vi "IMAQ Mask.vi"() -> ()   [LabVIEW 2012, in "LightPipes.lvlib"]
uses:
  LightPipes.lvlib
  <vilib>/vision/NI_Vision_Development_Module.lvlib
panel:
  in  "Image Type":u32(ring)=1 items=["8 bits", "16 bits", "Float", "Complex", "RGB", "HSL"]
  in  "Noise Value":i32
  in  "Noise Remove":bool
  in  "Save":bool
  in  "Input Image Path":path
  out "Image":T1(plugin-control)
  in  "Stop":bool
  in  "Mask":bool
  out "Mask":T1(plugin-control)
  # "1. Select the Image File\n2. Select the Region of Interest (ROI)\n3. Press Mask\n4. Press Save to save the masked picture\n5. Press Return to exit"
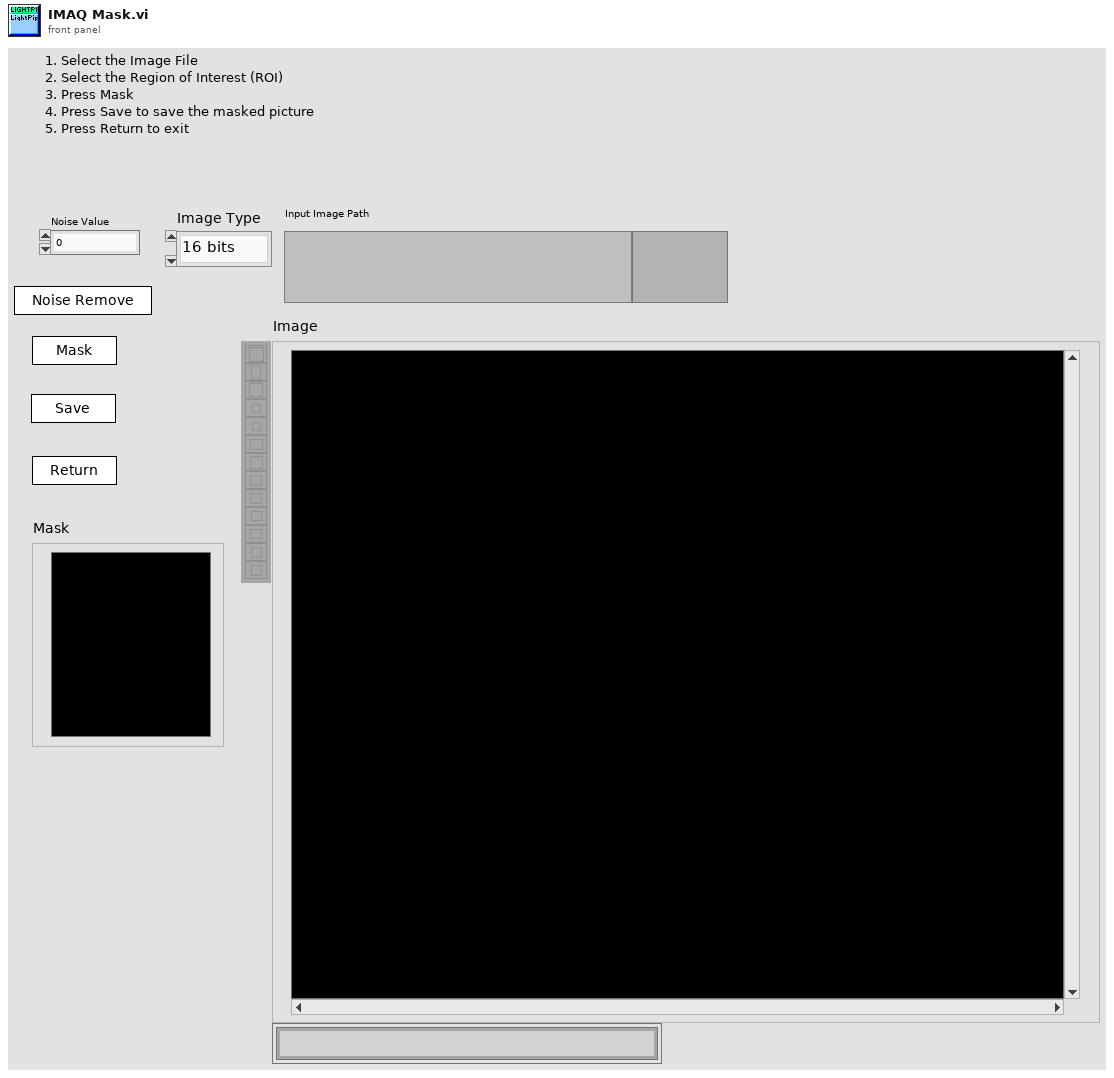
[diagram p1: front panel]
types:
  T1 = typedef "IMAQ Image.ctl" = refnum<image>
  T2 = cluster{"Global Rectangle":i32[], "Contours":cluster{"Contour Type":u32, "ROI Type":u32, "Points":i32[]}[]}
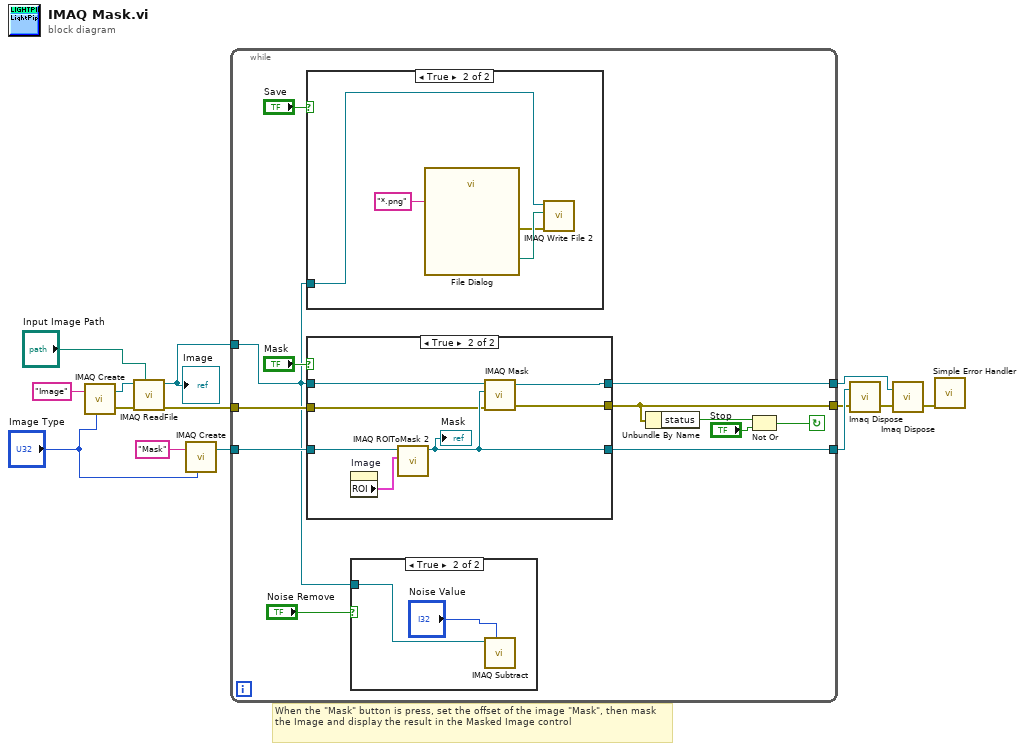
[diagram p0: block diagram]
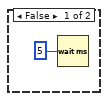
[diagram p3: hidden frame]
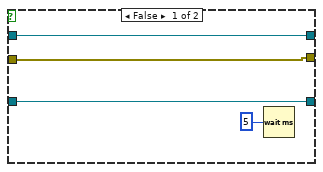
[diagram p4: hidden frame]
diagram:
  # "When the \"Mask\" button is press, set the offset of the image \"Mask\", then mask the Image and display the result in the Masked Image control"
  n1 = call "IMAQ Create"("Image Name"="Image", "Image Type"="Image Type") -> ("New Image"=w8:T1, "error out"=w13:errorcluster)  [unwired: 2 in, 1 out]
  n2 = call "IMAQ ReadFile"("File Path"="Input Image Path", "error in (no error)"=w13, "Image"=w8) -> ("error out"=w12:errorcluster, "Image Out"=w2:T1)  [unwired: 2 in, 5 out]
  "Image" <- w2
  n3 = call "IMAQ Create"("Image Name"="Mask", "Image Type"="Image Type") -> ("New Image"=w9:T1)  [unwired: 2 in, 2 out]
  n4 = while {
    tunnel: w2 -> [w15]
    tunnel: w12 -> [w25]
    tunnel: [w24] -> w3
    tunnel: [w18] -> w7
    tunnel: [w20] -> w5
    tunnel: w9 -> [w16]
    stop <- w21 continue-if-true
    n5 = case shown="True" "Save" {
      tunnel: w15 -> [_ w31]
      frame False {
        n6 = Wait (ms)(milliseconds to wait=u32 5) -> ()  [unwired: 1 out]
      }
      frame True {
        n7 = call "File Dialog"("pattern (all files)"="*.png") -> ("selected path"=w33:path, "error out"=w30:errorcluster)  [unwired: 11 in, 2 out]
        n8 = call-poly "IMAQ Write File 2"("error in (no error)"=w30, "File Path"=w33, "Image"=w31) -> ()  [unwired: 7 in, 2 out]
      }
    }
    n9 = case shown="True" "Mask" {
      tunnel: w15 -> [w37 w44]
      tunnel: w25 -> [w36 w40]
      tunnel: [w37 w38] -> w18
      tunnel: [w36 w43] -> w24
      tunnel: [w34 w41] -> w20
      tunnel: w16 -> [w34 w39]
      frame False {
        n10 = Wait (ms)(milliseconds to wait=u32 5) -> ()  [unwired: 1 out]
      }
      frame True {
        n11 = property on="Image" class="ImageControl"() -> ("ROI"=w42:T2)  [unwired: 2 in, 2 out]
        n12 = call "IMAQ ROIToMask 2"("ROI Descriptor"=w42, "Image"=w39) -> ("Image Out"=w41:T1)  [unwired: 7 in, 2 out]
        "Mask" <- w41
        n13 = call "IMAQ Mask"("error in (no error)"=w40, "Image Mask"=w41, "Image Src"=w44) -> ("error out"=w43:errorcluster, "Image Dst Out"=w38:T1)  [unwired: 1 in, 1 out]
      }
    }
    n14 = case shown="True" "Noise Remove" {
      tunnel: w15 -> [_ w28]
      frame False {
      }
      frame True {
        n15 = call "IMAQ Subtract"("Image Src A"=w28, "Constant"="Noise Value") -> ()  [unwired: 5 in, 2 out]
      }
    }
    n16 = Unbundle By Name(w24) -> ("status"=w23:bool)
    n17 = Not Or(1:"Stop", 2:w23) -> (0:w21:bool)
  }
  n18 = call "Imaq Dispose"("Image"=w5, "error in (no error)"=w3) -> ("error out"=w4:errorcluster)  [unwired: 1 in, 3 out]
  n19 = call "Imaq Dispose"("Image"=w7, "error in (no error)"=w4) -> ("error out"=w6:errorcluster)  [unwired: 1 in, 3 out]
  n20 = call <vilib>:"Simple Error Handler.vi"("error in (no error)"=w6) -> ()  [unwired: 1 in, 8 out]
